vi "多列列表框变换颜色.vi"(6 "奇数行字体颜色":u32(colorbox)=6618880, 7 "偶数行字体颜色":u32(colorbox)=16731648, 8 "error in":errorcluster, 9 "奇数行背景颜色":u32(colorbox)=11121611, 10 "偶数行背景颜色":u32(colorbox)=16777238, 11 "MCListbox Refnum in":refnum<vi>) -> (0 "error out":errorcluster, 3 "MCListbox Refnum out":refnum<vi>)   [LabVIEW 2015]
uses:
  <vilib>/Utility/miscctls.llb/LVRowAndColumnTypeDef.ctl
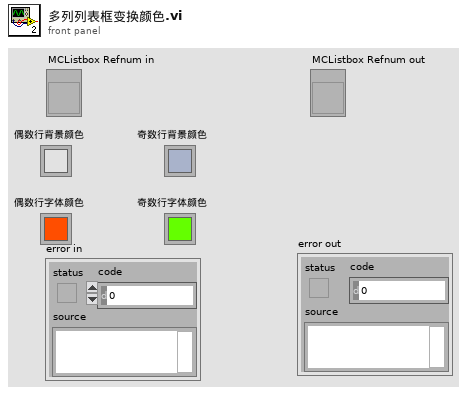
[diagram p1: front panel]
types:
  T1 = typedef "LVRowAndColumnTypeDef.ctl" = cluster{"Row":i32, "Column":i32}
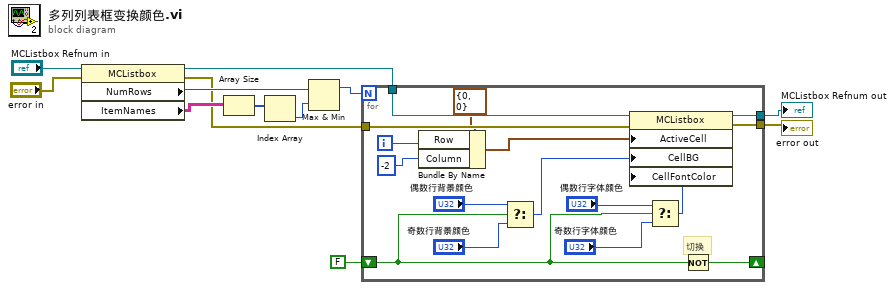
[diagram p0: block diagram]
diagram:
  n1 = property on="Property Node" class="MCListbox"(reference="MCListbox Refnum in", error in="error in") -> (reference out=w8:refnum<vi>, error out=w2:errorcluster, "NumRows"=w5:u32, "ItemNames"=w7:string[][])
  n2 = Array Size(array=w7) -> (size(s)=w6:i32[])
  n3 = Index Array(array=w6) -> (element=w4:i32)  [unwired: 1 in]
  n4 = Max & Min(x=w5, y=w4) -> (max(x,y)=w3:u32)  [unwired: 1 out]
  n5 = for {
    N: w3 -> [_]
    tunnel: w2 -> [w25]
    shift-right: [w28] -> _
    shift-left: FALSE -> [w20]
    tunnel: w8 -> [w16]
    tunnel: [w26] -> w9
    tunnel: [w24] -> w10
    i -> [w14]
    # "切换"
    n6 = Bundle By Name(cluster=T1 {"Row"=0, "Column"=0} ("Active Cell"), "Row"=w14, "Column"=-2) -> (w27:T1)
    n7 = Select(t="偶数行背景颜色", s=w20, f="奇数行背景颜色") -> (s? t:f=w21:u32)
    n8 = Select(t="偶数行字体颜色", s=w20, f="奇数行字体颜色") -> (s? t:f=w17:u32)
    n9 = property on="Property Node" class="MCListbox"(reference=w16, error in=w25, "ActiveCell"=w27, "CellBG"=w21, "CellFontColor"=w17) -> (reference out=w26:refnum<vi>, error out=w24:errorcluster)
    n10 = Not(x=w20) -> (.not. x?=w28:bool)
  }
  "error out" <- w10
  "MCListbox Refnum out" <- w9
